vi "ConfigureTrig.vi"(8 "error in (no error)":errorcluster, 10 "TrigName":string, 11 "SyncPluginBase in":refnum<class "SyncPluginBase.lvclass">) -> (0 "error out":errorcluster, 3 "SyncPluginBase out":refnum<class "SyncPluginBase.lvclass">)   [LabVIEW 2014, in "SyncPlugins.lvlib" / "SyncPluginBase.lvclass"]
uses:
  SyncPluginBase.lvclass
  <userlib>/NIST/BaseClasses/Object_class/BaseObject.lvclass
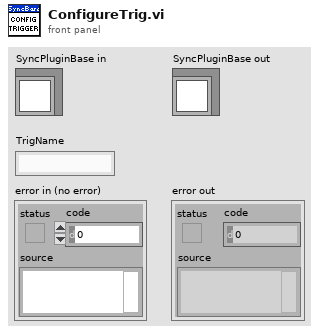
[diagram p1: front panel]
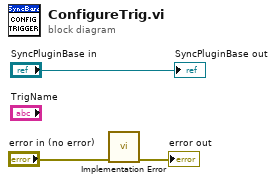
[diagram p0: block diagram]
diagram:
  n1 = call <userlib>:"Implementation Error.vi"("error in (no error)"="error in (no error)") -> ("error out"=→"error out":errorcluster)  [unwired: 10 in]
  "SyncPluginBase out" <- "SyncPluginBase in"
